vi "Message - Confirm Leakage.vi"(8 "error in":errorcluster) -> (0 "error out":errorcluster, 3 "OPTION":i32)   [LabVIEW 2014]
panel:
  out "STOP":bool
  in  "OPT3":bool caption="LEAKAGE DETECTED, STOP PROCESS."
  in  "OPT2":bool caption="LEAKAGE DETECTED, CHECK AGAIN."
  in  "OPT1":bool caption="NO LEAKAGE, CONTINUE PROCESS."
  in  "CONFIRM":bool
  # "CHECK LEAKAGE FROM \nINSPECTION CAMERA"
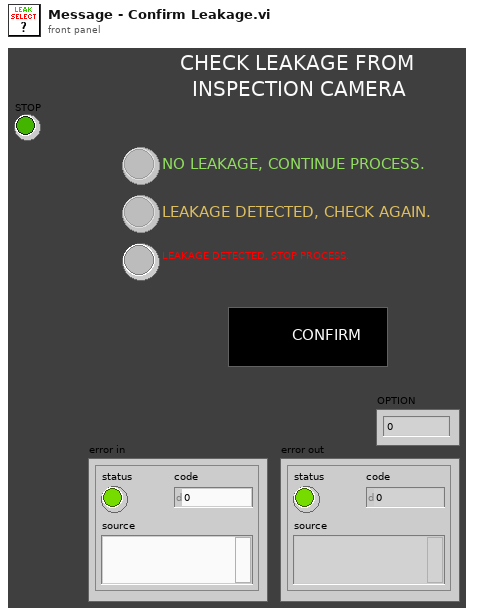
[diagram p1: front panel]
types:
  T1 = enum8{"Enabled", "Disabled", "Disabled and Grayed Out"}
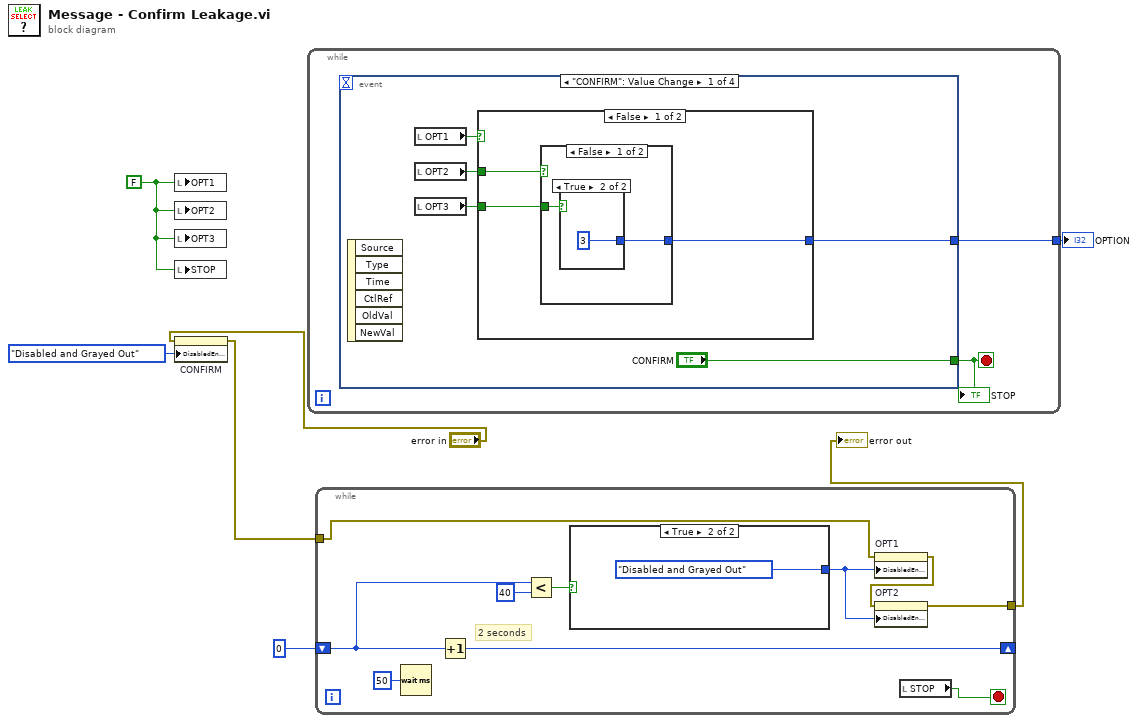
[diagram p0: block diagram]
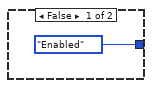
[diagram p2: hidden frame]
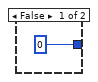
[diagram p3: hidden frame]
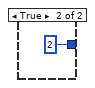
[diagram p4: hidden frame]
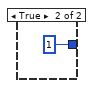
[diagram p5: hidden frame]
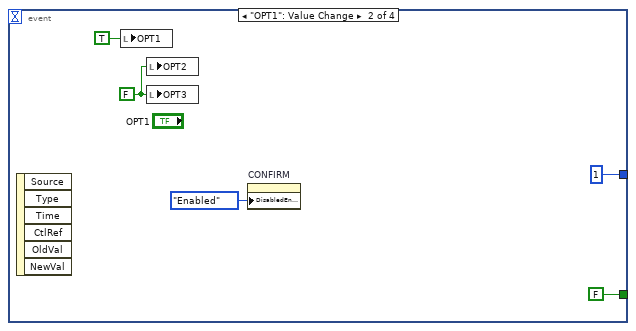
[diagram p6: hidden frame]
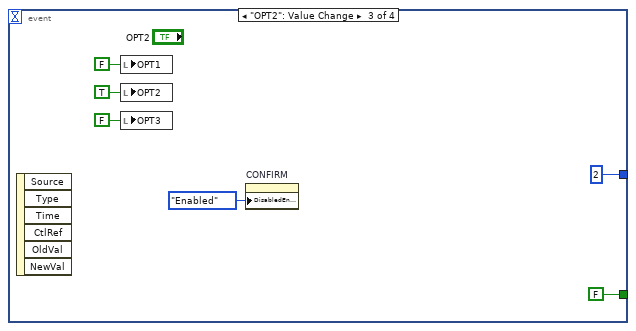
[diagram p7: hidden frame]
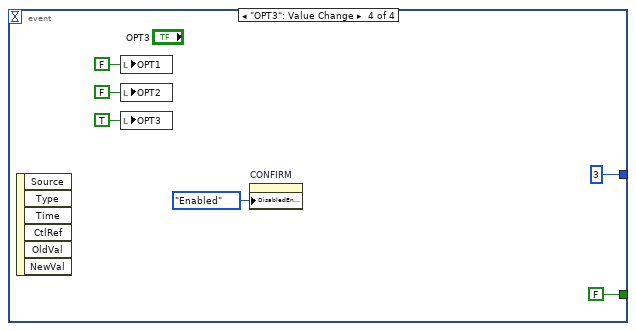
[diagram p8: hidden frame]
diagram:
  w1 = FALSE
  n1 = local write "OPT1"(w1) -> ()
  n2 = local write "OPT2"(w1) -> ()
  n3 = local write "OPT3"(w1) -> ()
  n4 = local write "STOP"(w1) -> ()
  n5 = property on="CONFIRM" class="Bool"(error in="error in", "DisabledEnum"=T1."Disabled and Grayed Out" ("Disabled")) -> (error out=w4:errorcluster)  [unwired: 1 in, 1 out]
  n6 = while {
    tunnel: [w9] -> w7
    stop <- w8 stop-if-true
    n7 = event shown="[0] \"CONFIRM\": Value Change" {
      selector: _ -> [_ _ _ _]
      dyn-events: _ -> [_ _ _ _]
      timeout: _ -> [_ _ _ _]
      tunnel: ["CONFIRM" FALSE ("CONFIRM") FALSE ("CONFIRM") FALSE ("CONFIRM")] -> w8
      tunnel: [w10 1 2 3] -> w9
      event "CONFIRM": Value Change {
        n8 = event-data() -> ()  [unwired: 1 in, 6 out]
        n9 = local read "OPT1"() -> (w13:bool)
        n10 = local read "OPT2"() -> (w12:bool)
        n11 = local read "OPT3"() -> (w11:bool)
        n12 = case shown="False" w13 {
          tunnel: w12 -> [w17 _]
          tunnel: w11 -> [w16 _]
          tunnel: [w15 1] -> w10
          frame False {
            n13 = case shown="False" w17 {
              tunnel: w16 -> [w19 _]
              tunnel: [w18 2] -> w15
              frame False {
                n14 = case shown="True" w19 {
                  tunnel: [0 3] -> w18
                  frame False {
                  }
                  frame True {
                  }
                }
              }
              frame True {
              }
            }
          }
          frame True {
          }
        }
      }
      event "OPT1": Value Change {
        w26 = FALSE ("OPT2")
        n15 = event-data() -> ()  [unwired: 1 in, 6 out]
        n16 = local write "OPT1"(TRUE ("OPT1")) -> ()
        n17 = local write "OPT2"(w26) -> ()
        n18 = local write "OPT3"(w26) -> ()
        n19 = property on="CONFIRM" class="Bool"("DisabledEnum"=T1."Enabled" ("Disabled")) -> ()  [unwired: 2 in, 2 out]
      }
      event "OPT2": Value Change {
        n20 = event-data() -> ()  [unwired: 1 in, 6 out]
        n21 = local write "OPT1"(FALSE ("OPT1")) -> ()
        n22 = local write "OPT2"(TRUE ("OPT2")) -> ()
        n23 = local write "OPT3"(FALSE ("OPT3")) -> ()
        n24 = property on="CONFIRM" class="Bool"("DisabledEnum"=T1."Enabled" ("Disabled")) -> ()  [unwired: 2 in, 2 out]
      }
      event "OPT3": Value Change {
        n25 = event-data() -> ()  [unwired: 1 in, 6 out]
        n26 = local write "OPT1"(FALSE ("OPT1")) -> ()
        n27 = local write "OPT2"(FALSE ("OPT2")) -> ()
        n28 = local write "OPT3"(TRUE ("OPT3")) -> ()
        n29 = property on="CONFIRM" class="Bool"("DisabledEnum"=T1."Enabled" ("Disabled")) -> ()  [unwired: 2 in, 2 out]
      }
    }
    "STOP" <- w8
  }
  "OPTION" <- w7
  n30 = while {
    shift-right: [w41] -> _
    shift-left: u32 0 ("milliseconds to wait") -> [w46]
    tunnel: w4 -> [w44]
    tunnel: [w43] -> w3
    stop <- w42 stop-if-true
    # "2 seconds"
    n31 = Wait (ms)(milliseconds to wait=u32 50) -> ()  [unwired: 1 out]
    n32 = Increment(x=w46) -> (x+1=w41:u32)
    n33 = Less?(x=w46, y=u32 40) -> (x < y?=w50:bool)
    n34 = case shown="True" w50 {
      tunnel: [T1."Enabled" ("Disabled") T1."Disabled and Grayed Out" ("Disabled")] -> w49
      frame False {
      }
      frame True {
      }
    }
    n35 = property on="OPT1" class="Bool (strict)"(error in=w44, "DisabledEnum"=w49) -> (error out=w48:errorcluster)  [unwired: 1 in, 1 out]
    n36 = property on="OPT2" class="Bool (strict)"(error in=w48, "DisabledEnum"=w49) -> (error out=w43:errorcluster)  [unwired: 1 in, 1 out]
    n37 = local read "STOP"() -> (w42:bool)
  }
  "error out" <- w3
